vi "ShortcutMenu.vi"(8 "error in":errorcluster, 9 "menu ref in":refnum<k9>, 11 "node in":refnum<class "sbRIO-9651.lvclass">) -> (0 "error out":errorcluster, 1 "menu ref out":refnum<k9>, 3 "node out":refnum<class "sbRIO-9651.lvclass">)   [LabVIEW 2014, in "sbRIO-9651.lvclass"]
doc: "Defines the behavior of the shortcut menu of the node."
uses:
  sbRIO-9651.lvclass
  RIO Target/RIO Target.lvclass
  <vilib>/NI/Configuration Framework/Node/NISE_CEF_Node.lvclass
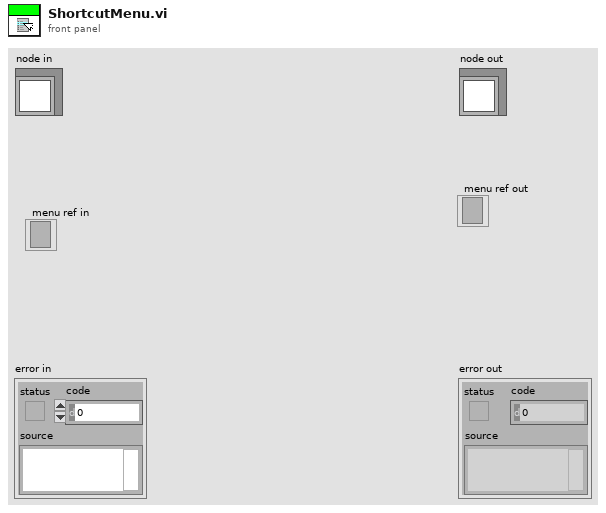
[diagram p1: front panel]
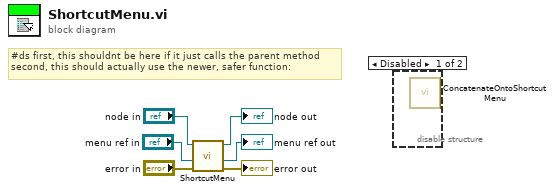
[diagram p0: block diagram]
diagram:
  # "#ds first, this shouldnt be here if it just calls the parent method\nsecond, this should actually use the newer, safer function:"
  n1 = call-parent "ShortcutMenu.vi"("error in"="error in", "menu ref in"="menu ref in", "node in"="node in") -> ("error out"=→"error out":errorcluster, "menu ref out"=→"menu ref out":refnum<k9>, "node out"=→"node out":refnum<class "sbRIO-9651.lvclass">)  [unwired: 6 in]
  n2 = disable-structure shown="Disabled" {
    frame Disabled {
      n3 = call-dynamic "ConcatenateOntoShortcutMenu.vi"() -> ()  [unwired: 9 in, 3 out]
    }
    frame Enabled {
    }
  }
